vi "set file meta.vi"(8 "error in (no error)":errorcluster, 11 "5785_2_x_1600MHz in":refnum<class "5785_2_x_1600MHz.lvclass">) -> (0 "error out":errorcluster, 3 "5785_2_x_1600MHz out":refnum<class "5785_2_x_1600MHz.lvclass">)   [LabVIEW 2021, in "5785_2_x_1600MHz.lvclass"]
uses:
  5785_2_x_1600MHz.lvclass
  5785_2_x_1600MHz.lvclass/5785_2_x_1600MHz.ctl
  pulse_tx_vis/CTL/device_mode.ctl
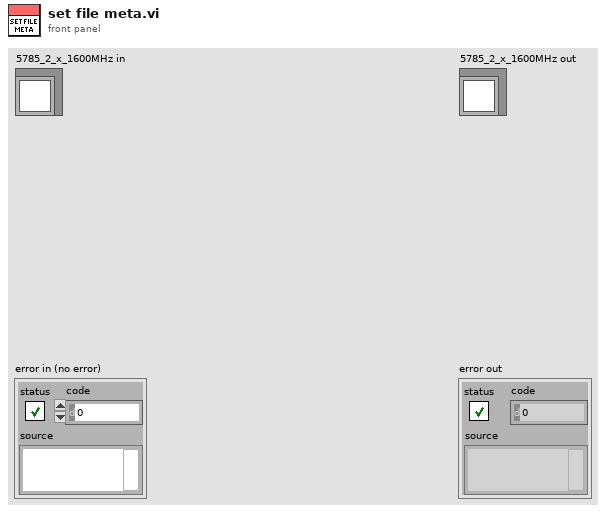
[diagram p1: front panel]
types:
  T1 = typedef "device_mode.ctl" = enum16{"USRP - 180MHz", "5785 - 2*180MHz", "5785 - 3.2GHz", "P2P - VST", "5785 2*1.6GHz"}
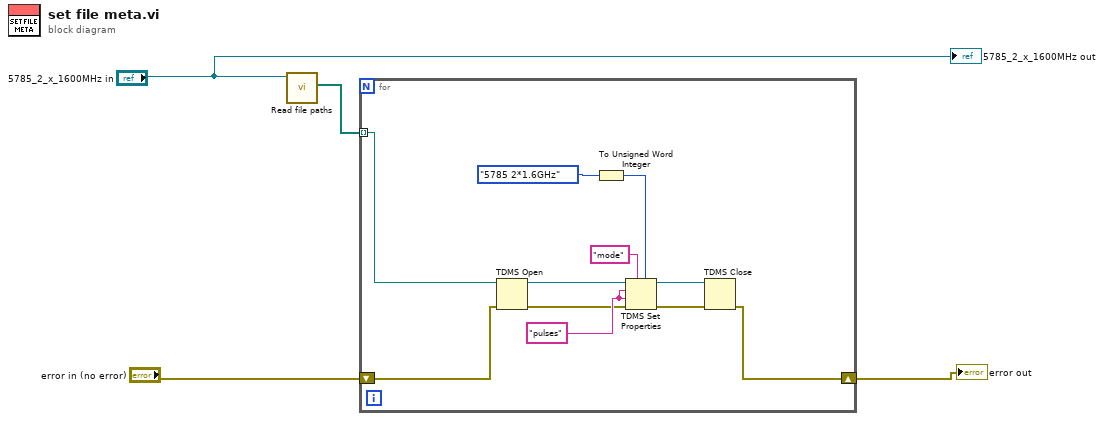
[diagram p0: block diagram]
diagram:
  n1 = call-dynamic "Read file paths.vi"("device_type in"="5785_2_x_1600MHz in") -> ("file paths"=w4:path[])  [unwired: 8 in, 2 out]
  n2 = for {
    tunnel: w4 -> [w13] mode=indexing
    shift-right: [w5] -> w1
    shift-left: "error in (no error)" -> [w6]
    w15 = "pulses" ("channel name")
    n3 = TDMS Open(8:w6, 11:w13) -> (0:w10:errorcluster, 3:w14:refnum<k34>)  [unwired: 5 in]
    n4 = To Unsigned Word Integer(number=device_mode."5785 2*1.6GHz" ("Mode")) -> (unsigned 16bit integer=w7:u16)
    n5 = TDMS Set Properties(5:w7, 7:"mode", 8:w10, 9:w15, 10:w15, 11:w14) -> (0:w11:errorcluster, 3:w12:refnum<k34>)  [unwired: 2 out]
    n6 = TDMS Close(8:w11, 11:w12) -> (0:w5:errorcluster)  [unwired: 1 out]
  }
  "error out" <- w1
  "5785_2_x_1600MHz out" <- "5785_2_x_1600MHz in"
